vi "GetPrice.vi"(8 "error in (no error)":errorcluster, 11 "Couch in":refnum<class "Couch.lvclass">) -> (0 "error out":errorcluster, 2 "Price":dbl, 3 "Couch out":refnum<class "Couch.lvclass">)   [LabVIEW 2019, in "Couch.lvclass"]
uses:
  Couch.lvclass
  Furniture.lvclass
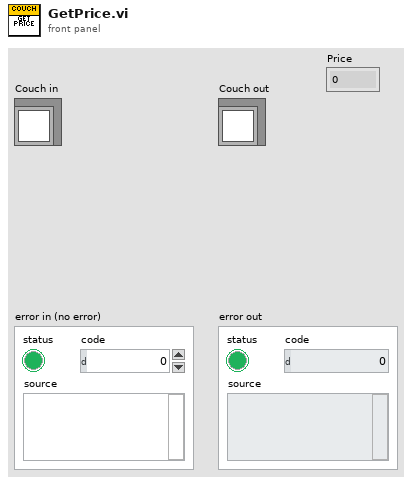
[diagram p1: front panel]
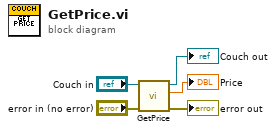
[diagram p0: block diagram]
diagram:
  n1 = call-parent "GetPrice.vi"("error in (no error)"="error in (no error)", "Furniture in"="Couch in") -> ("error out"=→"error out":errorcluster, "Price"=→"Price":dbl, "Furniture out"=→"Couch out":refnum<class "Couch.lvclass">)  [unwired: 7 in]
